vi "Auto Lift.vi"(11 "elevatorSpeed":dbl format="%#_13g") -> ()   [LabVIEW 2017]
uses:
  Common Code/Elevator Mode.ctl
  Robot Global Data.vi
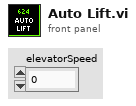
[diagram p1: front panel]
types:
  T1 = typedef "Elevator Mode.ctl" = enum16{"Semi Auto", "Manual", "Auto"}
  T2 = typedef "Elevator Command Cluster.ctl" = cluster{"Elevator Mode":T1, "Elevator State":T3, "Manual Speed":dbl, "Reset Encoders":bool, "High?":bool}
  T3 = typedef "Elevator State.ctl" = enum16{"Idle", "Ground", "Mid", "Scale", "Switch"}
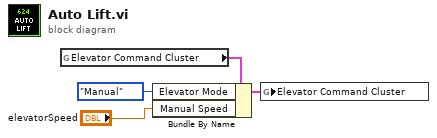
[diagram p0: block diagram]
diagram:
  n1 = global read "Robot Global Data.vi" "Elevator Command Cluster"() -> (w4:T2)
  n2 = Bundle By Name(cluster=w4, "Elevator Mode"=Elevator_Mode."Manual", "Manual Speed"="elevatorSpeed") -> (w3:T2)
  n3 = global write "Robot Global Data.vi" "Elevator Command Cluster"(w3) -> ()
